vi "polling_events.vi"() -> ()   [LabVIEW 2019]
uses:
  vi.lib/addons/zeromq/socket_type.ctl
  vi.lib/addons/zeromq/socket_options.ctl
  vi.lib/addons/zeromq/zmq_context.lvclass
  vi.lib/addons/zeromq/zeromq.lvlib
  vi.lib/addons/zeromq/zmq_socket.lvclass
panel:
  out "messages":string[](array[string])
  in  "endpoint":string="tcp://127.0.0.1:5555"
  # "ZeroMQ polling-based receive events"
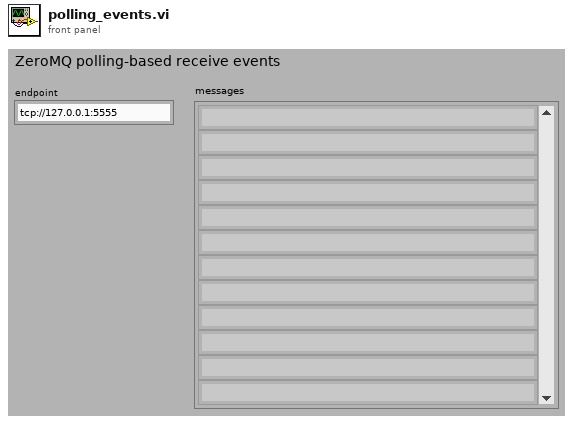
[diagram p1: front panel]
types:
  T1 = typedef "zeromq.lvlib/socket_options.ctl" = enum8{"NONE", "ZMQ_HWM", "<2>", "ZMQ_SWAP", "ZMQ_AFFINITY", "ZMQ_IDENTITY", "ZMQ_SUBSCRIBE", "ZMQ_UNSUBSCRIBE", "ZMQ_RATE", "ZMQ_RECOVERY_IVL", "ZMQ_MCAST_LOOP", "ZMQ_SNDBUF", "ZMQ_RCVBUF", "ZMQ_RCVMORE", "ZMQ_FD", "ZMQ_EVENTS", "ZMQ_TYPE", "ZMQ_LINGER", "ZMQ_RECONNECT_IVL", "ZMQ_BACKLOG", "ZMQ_RECOVERY_IVL_MSEC", "ZMQ_RECONNECT_IVL_MAX", "ZMQ_MAXMSGSIZE", "ZMQ_SNDHWM", "ZMQ_RCVHWM", "ZMQ_MULTICAST_HOPS", "<26>", "ZMQ_RCVTIMEO", "ZMQ_SNDTIMEO", "<29>", "<30>", "ZMQ_IPV4ONLY", "ZMQ_LAST_ENDPOINT", "ZMQ_ROUTER_MANDATORY", "ZMQ_TCP_KEEPALIVE", "ZMQ_TCP_KEEPALIVE_CNT", "ZMQ_TCP_KEEPALIVE_IDLE", "ZMQ_TCP_KEEPALIVE_INTVL", "ZMQ_TCP_ACCEPT_FILTER", "ZMQ_DELAY_ATTACH_ON_CONNECT", "ZMQ_XPUB_VERBOSE"}
  T2 = typedef "zeromq.lvlib/socket_type.ctl" = enum8{"ZMQ_PAIR", "ZMQ_PUB", "ZMQ_SUB", "ZMQ_REQ", "ZMQ_REP", "ZMQ_DEALER", "ZMQ_ROUTER", "ZMQ_PULL", "ZMQ_PUSH", "ZMQ_XPUB", "ZMQ_XSUB"}
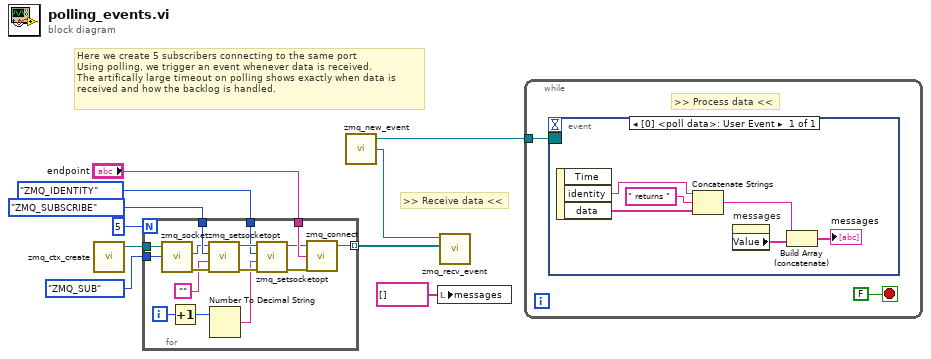
[diagram p0: block diagram]
diagram:
  # "Here we create 5 subscribers connecting to the same port\nUsing polling, we trigger an event whenever data is received.\nThe artifically large timeout on polling shows exactly when data is\nreceived and how the backlog is handled."
  # ">> Receive data <<"
  n1 = call "zmq_ctx_create.vi"() -> ("context out"=w10:refnum<class "zmq_context.lvclass">)  [unwired: 4 in, 1 out]
  n2 = for {
    N: 5 -> [_]
    tunnel: w10 -> [w26]
    tunnel: [w25] -> w4 mode=indexing
    tunnel: socket_options."ZMQ_SUBSCRIBE" ("option") -> [w23]
    tunnel: socket_type."ZMQ_SUB" ("socket type") -> [w22]
    tunnel: "endpoint" -> [w21]
    tunnel: socket_options."ZMQ_IDENTITY" ("option") -> [w14]
    i -> [w13]
    n3 = call "zmq_socket.vi"("socket type"=w22, "context in"=w26) -> ("error out"=w24:errorcluster, "socket out"=w20:refnum<class "zmq_socket.lvclass">)  [unwired: 3 in, 1 out]
    n4 = Increment(x=w13) -> (x+1=w11:i32)
    n5 = call "zmq_setsocketopt.vi"("error in"=w24, "value"="", "option"=w23, "socket in"=w20) -> ("error out"=w17:errorcluster, "socket out"=w18:refnum<class "zmq_socket.lvclass">)  [unwired: 2 in]
    n6 = Number To Decimal String(number=w11) -> (decimal integer string=w12:string)  [unwired: 1 in]
    n7 = call "zmq_setsocketopt.vi"("error in"=w17, "value"=w12, "option"=w14, "socket in"=w18) -> ("error out"=w16:errorcluster, "socket out"=w15:refnum<class "zmq_socket.lvclass">)  [unwired: 2 in]
    n8 = call "zmq_connect.vi"("error in"=w16, "endpoint"=w21, "socket in"=w15) -> ("socket out"=w25:refnum<class "zmq_socket.lvclass">)  [unwired: 1 in, 1 out]
  }
  n9 = call "zmq_new_event.vi"() -> ("user event"=w2:refnum<user-event>, "event ref out"=w3:refnum<event-registration>)  [unwired: 3 in, 1 out]
  n10 = local write "messages"(string[] [] ("messages")) -> ()
  n11 = call "zmq_recv_event.vi"("sockets"=w4, "poll event"=w2) -> ()  [unwired: 4 in, 2 out]
  n12 = while {
    tunnel: w3 -> [w28]
    stop <- FALSE stop-if-true
    # ">> Process data <<"
    n13 = event shown="[0] <poll data>: User Event" {
      selector: w28 -> [_]
      dyn-events: _ -> [_]
      timeout: _ -> [_]
      event User Event {
        n14 = event-data() -> ("identity"=w29:string, "data"=w30:string[])  [unwired: 1 in, 1 out]
        n15 = Concatenate Strings(w29, " returns " ("string"), w30) -> (w33:string)
        n16 = property on="messages" class="Arr (strict)"() -> ("Value"=w32:string[])  [unwired: 2 in, 2 out]
        n17 = Build Array (concatenate)(w33, w32) -> (→"messages":string[])
      }
    }
  }
